vi "RANGE ANSI Display.vi"(7 "Meter Number":T1, 8 "Error In":errorcluster, 9 "Elapsed Time":dbl, 11 "DAQ Data Out in":T2) -> (0 "Error Out":errorcluster, 3 "DAQ Data Out in 2":T2={"Meter 1"={"Meter Size"=0.0, "DAQ Output (Voltage)"=0.0, "Reference (Voltage)"=0.0, "Meter Present"=FALSE, "Meter Visa"="COM3", "Gas Type"="", "SLPM Error @ Zero"=0.0, "Gas Mix Number"="", "Set STP Register"=FALSE}, "Meter 2"={"Meter Size"=0.0, "DAQ Output (Voltage)"=0.0, "Reference (Voltage)"=0.0, "Meter Present"=FALSE, "Meter Visa"="COM4", "Gas Type"="", "SLPM Error @ Zero"=0.0, "Gas Mix Number"="", "Set STP Register"=FALSE}, "Meter 3"={"Meter Size"=0.0, "DAQ Output (Voltage)"=0.0, "Reference (Voltage)"=0.0, "Meter Present"=FALSE, "Meter Visa"="COM5", "Gas Type"="", "SLPM Error @ Zero"=0.0, "Gas Mix Number"="", "Set STP Register"=FALSE}, "Meter 4"={"Meter Size"=0.0, "DAQ Output (Voltage)"=0.0, "Reference (Voltage)"=0.0, "Meter Present"=FALSE, "Meter Visa"="COM6", "Gas Type"="", "SLPM Error @ Zero"=0.0, "Gas Mix Number"="", "Set STP Register"=FALSE}, "Meter 5"={"Meter Size"=0.0, "DAQ Output (Voltage)"=0.0, "Reference (Voltage)"=0.0, "Meter Present"=FALSE, "Meter Visa"="COM7", "Gas Type"="", "SLPM Error @ Zero"=0.0, "Gas Mix Number"="", "Set STP Register"=FALSE}, "Meter 6"={"Meter Size"=0.0, "DAQ Output (Voltage)"=0.0, "Reference (Voltage)"=0.0, "Meter Present"=FALSE, "Meter Visa"="COM8", "Gas Type"="", "SLPM Error @ Zero"=0.0, "Gas Mix Number"="", "Set STP Register"=FALSE}, "Meter Bank 1"={"Flow Rate (BTU/HR)"=0.0, "ANSI Placeholder Array"=[], "15 Sec Avg Array"=[], "30 Sec Avg Array "=[], "ANSI Average (BTU/HR)"=0.0, "Panel Data"={"Meter Type (Gas)"="", "Meter ID"=enum."Disabled", "Heating Value (BTU/ft³)"=0.0, "Ft³ / Hr (SCFH)"=0.0, "15 Second Average (BTU/HR)"=0.0, "30 Second Average (BTU/HR)"=0.0, "SLPM (Mass Flow)"=0.0, "LPM (Vol. Flow)"=0.0, "Gas Temperature (°F)"=0.0, "Gas Pressure (PSIA)"=0.0, "Tot.Flow (Liters)"=0.0}, "Start ANSI"=FALSE, "ANSI Start Time"=0.0, "Restart ANSI"=FALSE}, "Meter Bank 2"={"Flow Rate (BTU/HR)"=0.0, "ANSI Placeholder Array"=[], "15 Sec Avg Array"=[], "30 Sec Avg Array "=[], "ANSI Average (BTU/HR)"=0.0, "Panel Data"={"Meter Type (Gas)"="", "Meter ID"=enum."Disabled", "Heating Value (BTU/ft³)"=0.0, "Ft³ / Hr (SCFH)"=0.0, "15 Second Average (BTU/HR)"=0.0, "30 Second Average (BTU/HR)"=0.0, "SLPM (Mass Flow)"=0.0, "LPM (Vol. Flow)"=0.0, "Gas Temperature (°F)"=0.0, "Gas Pressure (PSIA)"=0.0, "Tot.Flow (Liters)"=0.0}, "Start ANSI"=FALSE, "ANSI Start Time"=0.0, "Restart ANSI"=FALSE}, "Meter Bank 3"={"Flow Rate (BTU/HR)"=0.0, "ANSI Placeholder Array"=[], "15 Sec Avg Array"=[], "30 Sec Avg Array "=[], "ANSI Average (BTU/HR)"=0.0, "Panel Data"={"Meter Type (Gas)"="", "Meter ID"=enum."Disabled", "Heating Value (BTU/ft³)"=0.0, "Ft³ / Hr (SCFH)"=0.0, "15 Second Average (BTU/HR)"=0.0, "30 Second Average (BTU/HR)"=0.0, "SLPM (Mass Flow)"=0.0, "LPM (Vol. Flow)"=0.0, "Gas Temperature (°F)"=0.0, "Gas Pressure (PSIA)"=0.0, "Tot.Flow (Liters)"=0.0}, "Start ANSI"=FALSE, "ANSI Start Time"=0.0, "Restart ANSI"=FALSE}, "Threshold Voltage (NI DAQ)"=0.2, "Use RS232 Data Collection"=FALSE})   [LabVIEW 2016]
uses:
  Type Definitions/RANGE DAQ Data Four Meters.ctl
  Type Definitions/RANGE DAQ Data.ctl
  Drivers/Omega FMA-1600A Series Gas Flow Meter/Type Definitions/FMA1600A Gas Type.ctl
  Type Definitions/RANGE GAS Data.ctl
  Type Definitions/RANGE Panel Data.ctl
  Type Definitions/RANGE Meter Selector 1-2.ctl
  Type Definitions/Range Meter Bank.ctl
panel:
  out "ANSI Average (BTU/hr)":dbl
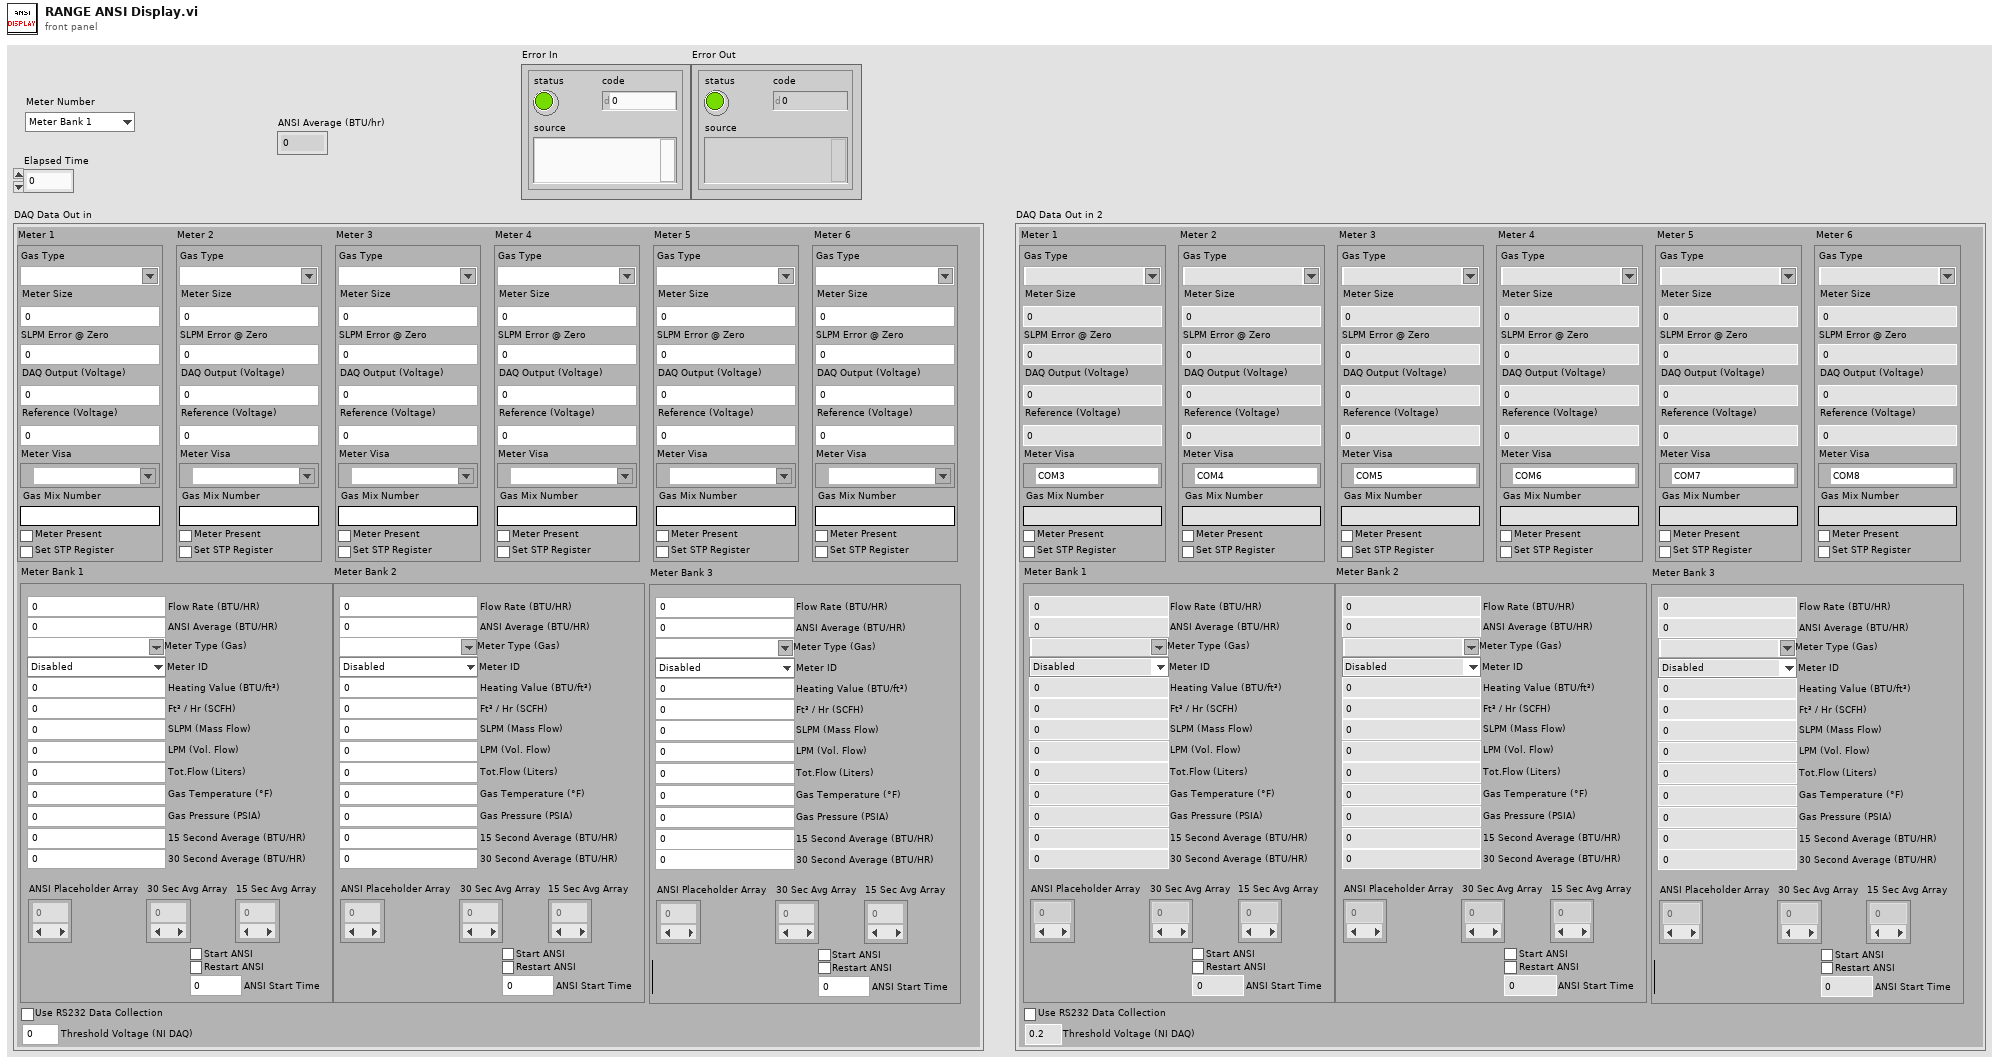
[diagram p1: front panel]
types:
  T1 = typedef "Range Meter Bank.ctl" = enum16{"Meter Bank 1", "Meter Bank 2", "Meter Bank 3"}
  T2 = typedef "RANGE DAQ Data Four Meters.ctl" = cluster{"Meter 1":T3, "Meter 2":T3, "Meter 3":T3, "Meter 4":T3, "Meter 5":T3, "Meter 6":T3, "Meter Bank 1":T5, "Meter Bank 2":T5, "Meter Bank 3":T5, "Threshold Voltage (NI DAQ)":dbl, "Use RS232 Data Collection":bool}
  T3 = typedef "RANGE DAQ Data.ctl" = cluster{"Meter Size":dbl, "DAQ Output (Voltage)":dbl, "Reference (Voltage)":dbl, "Meter Present":bool, "Meter Visa":refnum<visa-resource-name>, "Gas Type":T4, "SLPM Error @ Zero":dbl, "Gas Mix Number":string, "Set STP Register":bool}
  T4 = typedef "FMA1600A Gas Type.ctl" = string
  T5 = typedef "RANGE GAS Data.ctl" = cluster{"Flow Rate (BTU/HR)":dbl, "ANSI Placeholder Array":dbl[], "15 Sec Avg Array":dbl[], "30 Sec Avg Array ":dbl[], "ANSI Average (BTU/HR)":dbl, "Panel Data":T6, "Start ANSI":bool, "ANSI Start Time":dbl, "Restart ANSI":bool}
  T6 = typedef "RANGE Panel Data.ctl" = cluster{"Meter Type (Gas)":T4, "Meter ID":T7, "Heating Value (BTU/ft³)":dbl, "Ft³ / Hr (SCFH)":dbl, "15 Second Average (BTU/HR)":dbl, "30 Second Average (BTU/HR)":dbl, "SLPM (Mass Flow)":dbl, "LPM (Vol. Flow)":dbl, "Gas Temperature (°F)":dbl, "Gas Pressure (PSIA)":dbl, "Tot.Flow (Liters)":dbl}
  T7 = typedef "RANGE Meter Selector 1-2.ctl" = enum16{"Disabled", "Small", "Large"}
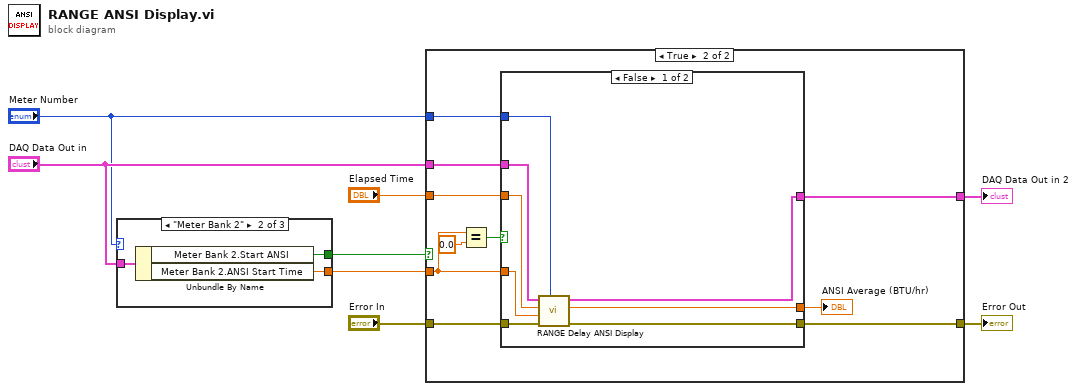
[diagram p0: block diagram]
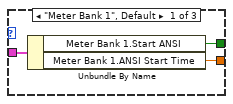
[diagram p2: hidden frame]
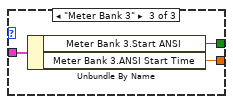
[diagram p3: hidden frame]
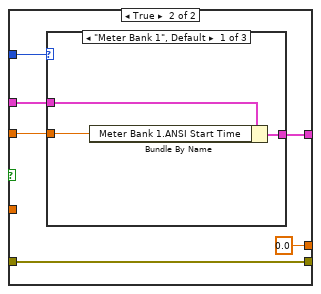
[diagram p5: hidden frame]
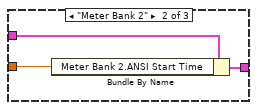
[diagram p6: hidden frame]
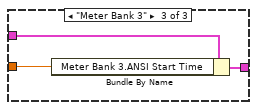
[diagram p7: hidden frame]
diagram:
  n1 = case shown="\"Meter Bank 2\"" "Meter Number" {
    tunnel: [w11 w12 w15] -> w8
    tunnel: [w10 w13 w16] -> w7
    tunnel: "DAQ Data Out in" -> [w9 w14 w17]
    frame "Meter Bank 1", Default {
      n2 = Unbundle By Name(w9) -> ("Meter Bank 1.Start ANSI"=w10:bool, "Meter Bank 1.ANSI Start Time"=w11:dbl)
    }
    frame "Meter Bank 2" {
      n3 = Unbundle By Name(w14) -> ("Meter Bank 2.Start ANSI"=w13:bool, "Meter Bank 2.ANSI Start Time"=w12:dbl)
    }
    frame "Meter Bank 3" {
      n4 = Unbundle By Name(w17) -> ("Meter Bank 3.Start ANSI"=w16:bool, "Meter Bank 3.ANSI Start Time"=w15:dbl)
    }
  }
  n5 = case shown="True" w7 {
    tunnel: "Elapsed Time" -> [_ w27]
    tunnel: "DAQ Data Out in" -> [w19 w26]
    tunnel: w8 -> [_ w25]
    tunnel: [w19 w24] -> w4
    tunnel: "Error In" -> [w18 w22]
    tunnel: [w18 w21] -> w2
    tunnel: "Meter Number" -> [_ w20]
    frame False {
    }
    frame True {
      n6 = Equal?(x=w25, y=0.0) -> (x = y?=w28:bool)
      n7 = case shown="False" w28 {
        tunnel: w27 -> [w36 w42]
        tunnel: w26 -> [w35 w43]
        tunnel: w25 -> [w37 _]
        tunnel: [w34 w41] -> w24
        tunnel: [w33 0.0] -> w23
        tunnel: w22 -> [w32 w39]
        tunnel: [w31 w39] -> w21
        tunnel: w20 -> [w30 w38]
        frame False {
          n8 = call "RANGE Delay ANSI Display.vi"("Meter Number"=w30, "Error In"=w32, "ANSI Start Time"=w37, "Elapsed Time"=w36, "DAQ Data Out in in"=w35) -> ("Error Out"=w31:errorcluster, "Display ANSI Average (BTU/hr) out"=w33:dbl, "DAQ Data Out out"=w34:T2)  [unwired: 4 in]
        }
        frame True {
          n9 = case shown="\"Meter Bank 1\", Default" w38 {
            tunnel: w43 -> [w46 w49 w52]
            tunnel: w42 -> [w45 w47 w50]
            tunnel: [w44 w48 w51] -> w41
            frame "Meter Bank 1", Default {
              n10 = Bundle By Name(cluster=w46, "Meter Bank 1.ANSI Start Time"=w45) -> (w44:T2)
            }
            frame "Meter Bank 2" {
              n11 = Bundle By Name(cluster=w49, "Meter Bank 2.ANSI Start Time"=w47) -> (w48:T2)
            }
            frame "Meter Bank 3" {
              n12 = Bundle By Name(cluster=w52, "Meter Bank 3.ANSI Start Time"=w50) -> (w51:T2)
            }
          }
        }
      }
      "ANSI Average (BTU/hr)" <- w23
    }
  }
  "Error Out" <- w2
  "DAQ Data Out in 2" <- w4
